vi "LVClass_HasoData Get Compute Phase Set.vi"(0 "HasoData in":refnum<class "HasoData.lvclass">, 5 "ComputePhaseSet in":refnum<class "ComputePhaseSet.lvclass">, 7 "ModalCoef in":refnum<class "ModalCoef.lvclass">, 11 "error in (no error)":errorcluster) -> (4 "HasoData out":refnum<class "HasoData.lvclass">, 6 "ComputePhaseSet out":refnum<class "ComputePhaseSet.lvclass">, 8 "ModalCoef out":refnum<class "ModalCoef.lvclass">, 15 "error out":errorcluster)   [LabVIEW 2020, in "HasoData.lvclass"]
doc: "Get ComputePhaseSet object.\n\n--------------------------------------------------------------------------------\n\n<B>HasoDataIn </B> : HasoData object.\n<B>HasoDataOut </B> : HasoData object.\n<B>ComputePhaseSet </B> : ComputePhaseSet object.\n<B>ErrorIn </B> : Error\n<B>ErrorOut </B> : Error\n\n--------------------------------------------------------------------------------"
uses:
  HasoData.lvclass
  ComputePhaseSet.lvclass
  ModalCoef.lvclass
  HasoData.lvclass/HasoData.ctl
  LVClass_ModalCoef Read ModalCoef.vi
  LVClass_ComputePhaseSet Read ComputePhaseSet.vi
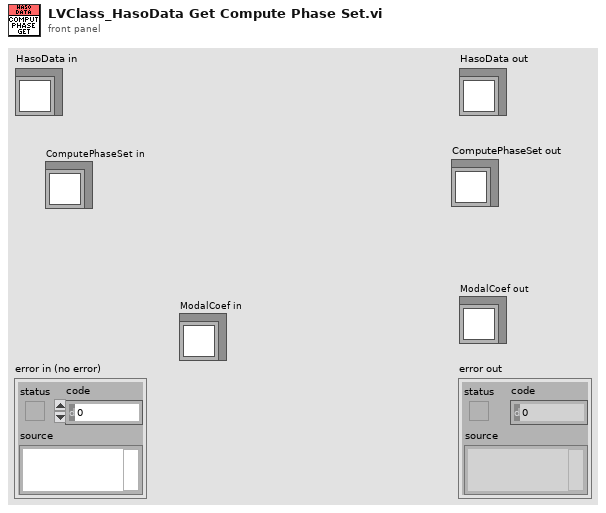
[diagram p1: front panel]
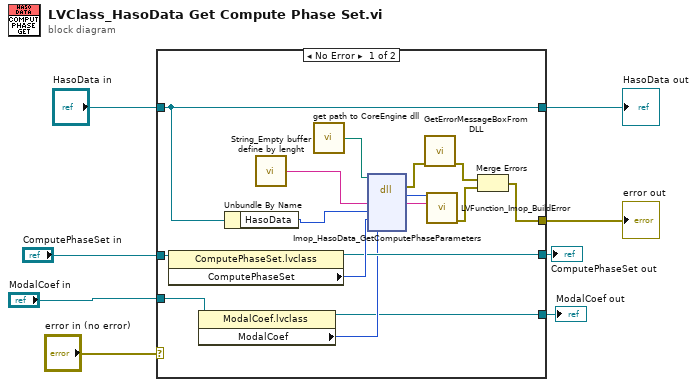
[diagram p0: block diagram]
diagram:
  n1 = case shown="No Error" "error in (no error)" {
    selector: "error in (no error)" -> [_ w28]
    tunnel: [w12 w28] -> w6
    tunnel: [w17 w27] -> w5
    tunnel: "HasoData in" -> [w17 w27]
    tunnel: "ComputePhaseSet in" -> [w19 w26]
    tunnel: [w15 w26] -> w3
    tunnel: "ModalCoef in" -> [w11 w25]
    tunnel: [w9 w25] -> w1
    frame No Error {
      n2 = property class="ComputePhaseSet.lvclass"(reference=w19) -> (reference out=w15:refnum<class "ComputePhaseSet.lvclass">, "ComputePhaseSet"=w18:i32)  [unwired: 1 in, 1 out]
      n3 = property class="ModalCoef.lvclass"(reference=w11) -> (reference out=w9:refnum<class "ModalCoef.lvclass">, "ModalCoef"=w10:u32)  [unwired: 1 in, 1 out]
      n4 = Unbundle By Name(w17) -> ("HasoData"=w16:i32)
      n5 = call "String_Empty buffer define by lenght.vi"() -> ("Empty buffer"=w22:string)  [unwired: 1 in]
      n6 = call "get path to CoreEngine dll.vi"() -> ("path to c_interface_vc100.dll"=w21:path)  [unwired: 12 in, 3 out]
      n7 = dll-call lib="D:/2_trunk/Soft_haso/ImOpCoreEngine4_LV2011/DLLs/ImopEngine4_vc100.dll" fn="Imop_HasoData_GetComputePhaseParameters"(path in=w21, "message"=w22, "objet"=w16, "ComputePhaseSet"=w18, "ModalCoef"=w10) -> (error out=w20:errorcluster, "return type"=w24:i32, "message"=w23:string)  [unwired: 5 in, 1 out]
      n8 = call "GetErrorMessageBoxFromDLL.vi"("error IN"=w20) -> ("error OUT"=w14:errorcluster)  [unwired: 10 in]
      n9 = call "LVFunction_Imop_BuildError.vi"("code"=w24, "String to Prepend to source (\"\")"=w23) -> ("error out"=w13:errorcluster)  [unwired: 13 in]
      n10 = Merge Errors(w14, w13) -> (w12:errorcluster)
    }
    frame Error {
    }
  }
  "error out" <- w6
  "HasoData out" <- w5
  "ComputePhaseSet out" <- w3
  "ModalCoef out" <- w1
